vi "GetSequence.vi"(7 "Num of Seq":i32, 8 "error in (no error)":errorcluster, 9 "actual  record length":i32, 10 "Channel name":string, 11 "inst handle IN":refnum<k15>) -> (0 "error out":errorcluster, 1 "initial x":dbl format="%.2f", 2 "x inc mics":dbl format="%.2f", 3 "inst handle OUT":refnum<k15>, 4 "waveform array":dbl[][](array[numeric]) format="%.2f", 6 "Actual Pts":i32)   [LabVIEW 2022 SP3]
panel:
  out "Att dB":dbl format="%.2f"
  out "Volt pp":dbl format="%.2f"
  out "V/ div":string
  out "Intensity Graph":dbl[][](graph)
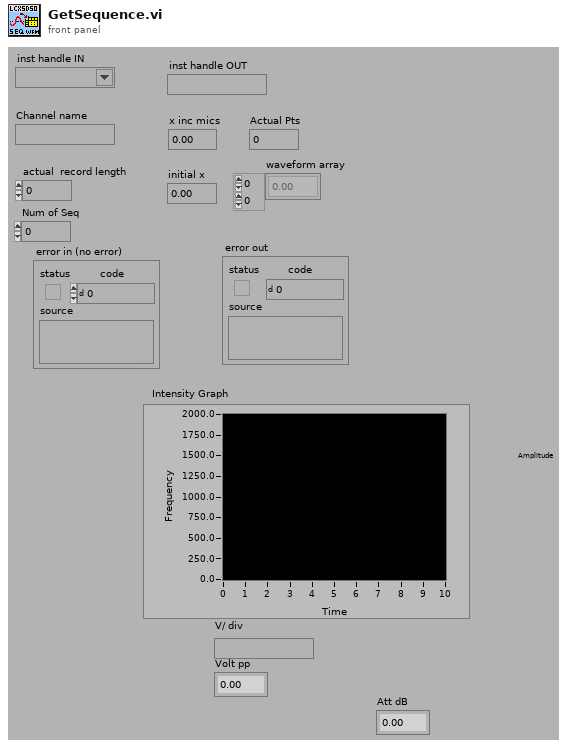
[diagram p1: front panel]
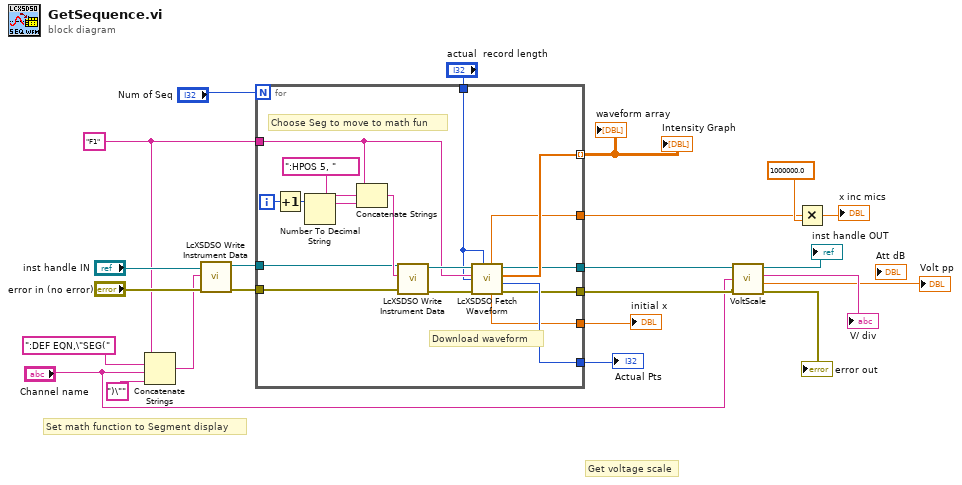
[diagram p0: block diagram]
diagram:
  w5 = "F1"
  # "Get voltage scale"
  # "Set math function to Segment display"
  n1 = Concatenate Strings(w5, ":DEF EQN,\"SEG(", "Channel name", ")\"") -> (w11:string)
  n2 = call "LcXSDSO Write Instrument Data.vi"("error in (no error)"="error in (no error)", "write buffer"=w11, "instrument handle"="inst handle IN") -> ("error out"=w15:errorcluster, "instrument handle out"=w14:refnum<k15>)  [unwired: 7 in]
  n3 = for {
    N: "Num of Seq" -> [_]
    tunnel: [w35] -> w9 mode=indexing
    tunnel: [w34] -> w23
    tunnel: [w33] -> w22
    tunnel: [w32] -> w8
    tunnel: [w31] -> w19
    tunnel: [w30] -> w7
    tunnel: w15 -> [w29]
    tunnel: w14 -> [w28]
    tunnel: w5 -> [w27]
    tunnel: "actual  record length" -> [w24]
    i -> [w26]
    # "Download waveform"
    # "Choose Seg to move to math fun"
    n4 = Increment(x=w26) -> (x+1=w25:i32)
    n5 = Number To Decimal String(number=w25) -> (decimal integer string=w39:string)  [unwired: 1 in]
    n6 = Concatenate Strings(w27, ":HPOS 5, ", w39) -> (w40:string)
    n7 = call "LcXSDSO Write Instrument Data.vi"("error in (no error)"=w29, "write buffer"=w40, "instrument handle"=w28) -> ("error out"=w36:errorcluster, "instrument handle out"=w37:refnum<k15>)  [unwired: 7 in]
    n8 = call "LcXSDSO Fetch Waveform.vi"("size of waveform array"=w24, "error in (no error)"=w36, "waveform size"=w24, "channel name"=w27, "instrument handle"=w37) -> ("error out"=w30:errorcluster, "actual points"=w34:i32, "waveform array"=w35:dbl[], "instrument handle out"=w32:refnum<k15>, "initial x"=w33:dbl, "x increment"=w31:dbl)  [unwired: 1 in]
  }
  "waveform array" <- w9
  "Actual Pts" <- w23
  "initial x" <- w22
  "Intensity Graph" <- w9
  n9 = call "VoltScale.vi"("instrument handle in"=w8, "Channel name"="Channel name", "error in"=w7) -> ("inst handle OUT"=→"inst handle OUT":refnum<k15>, "V/ div"=→"V/ div":string, "FS Volt pp"=→"Volt pp":dbl, "error out"=→"error out":errorcluster)  [unwired: 1 in]
  n10 = Multiply(x=w19, y=1000000.0) -> (x*y=→"x inc mics":dbl)
